vi "daqRead.vi"   [LabVIEW 2017]
doc: "From the DAQ card, reads into shared variables the external frame counter, the piezo monitor, and its differentiator. The acquisition is triggered by the Hamamatsu camera triggers. If daqSave is set to true, writes the values to file. \n\nThe acquisition loop stops with a daqStop (generally issued by the hamamatsuRead* VI) or, after a delay, with a generalStop."
uses:
  <vilib>/DAQmx/read.llb/DAQmx Read (Analog 1D DBL NChan 1Samp).vi
  <vilib>/DAQmx/read.llb/DAQmx Read (Counter U32 1Chan 1Samp).vi
  globalDevices.vi
  globalUtilities.vi
  <vilib>/DAQmx/miscellaneous.llb/DAQmx Fill In Error Info.vi
  <vilib>/DAQmx/read.llb/DAQmx Read (Analog DBL 1Chan 1Samp).vi
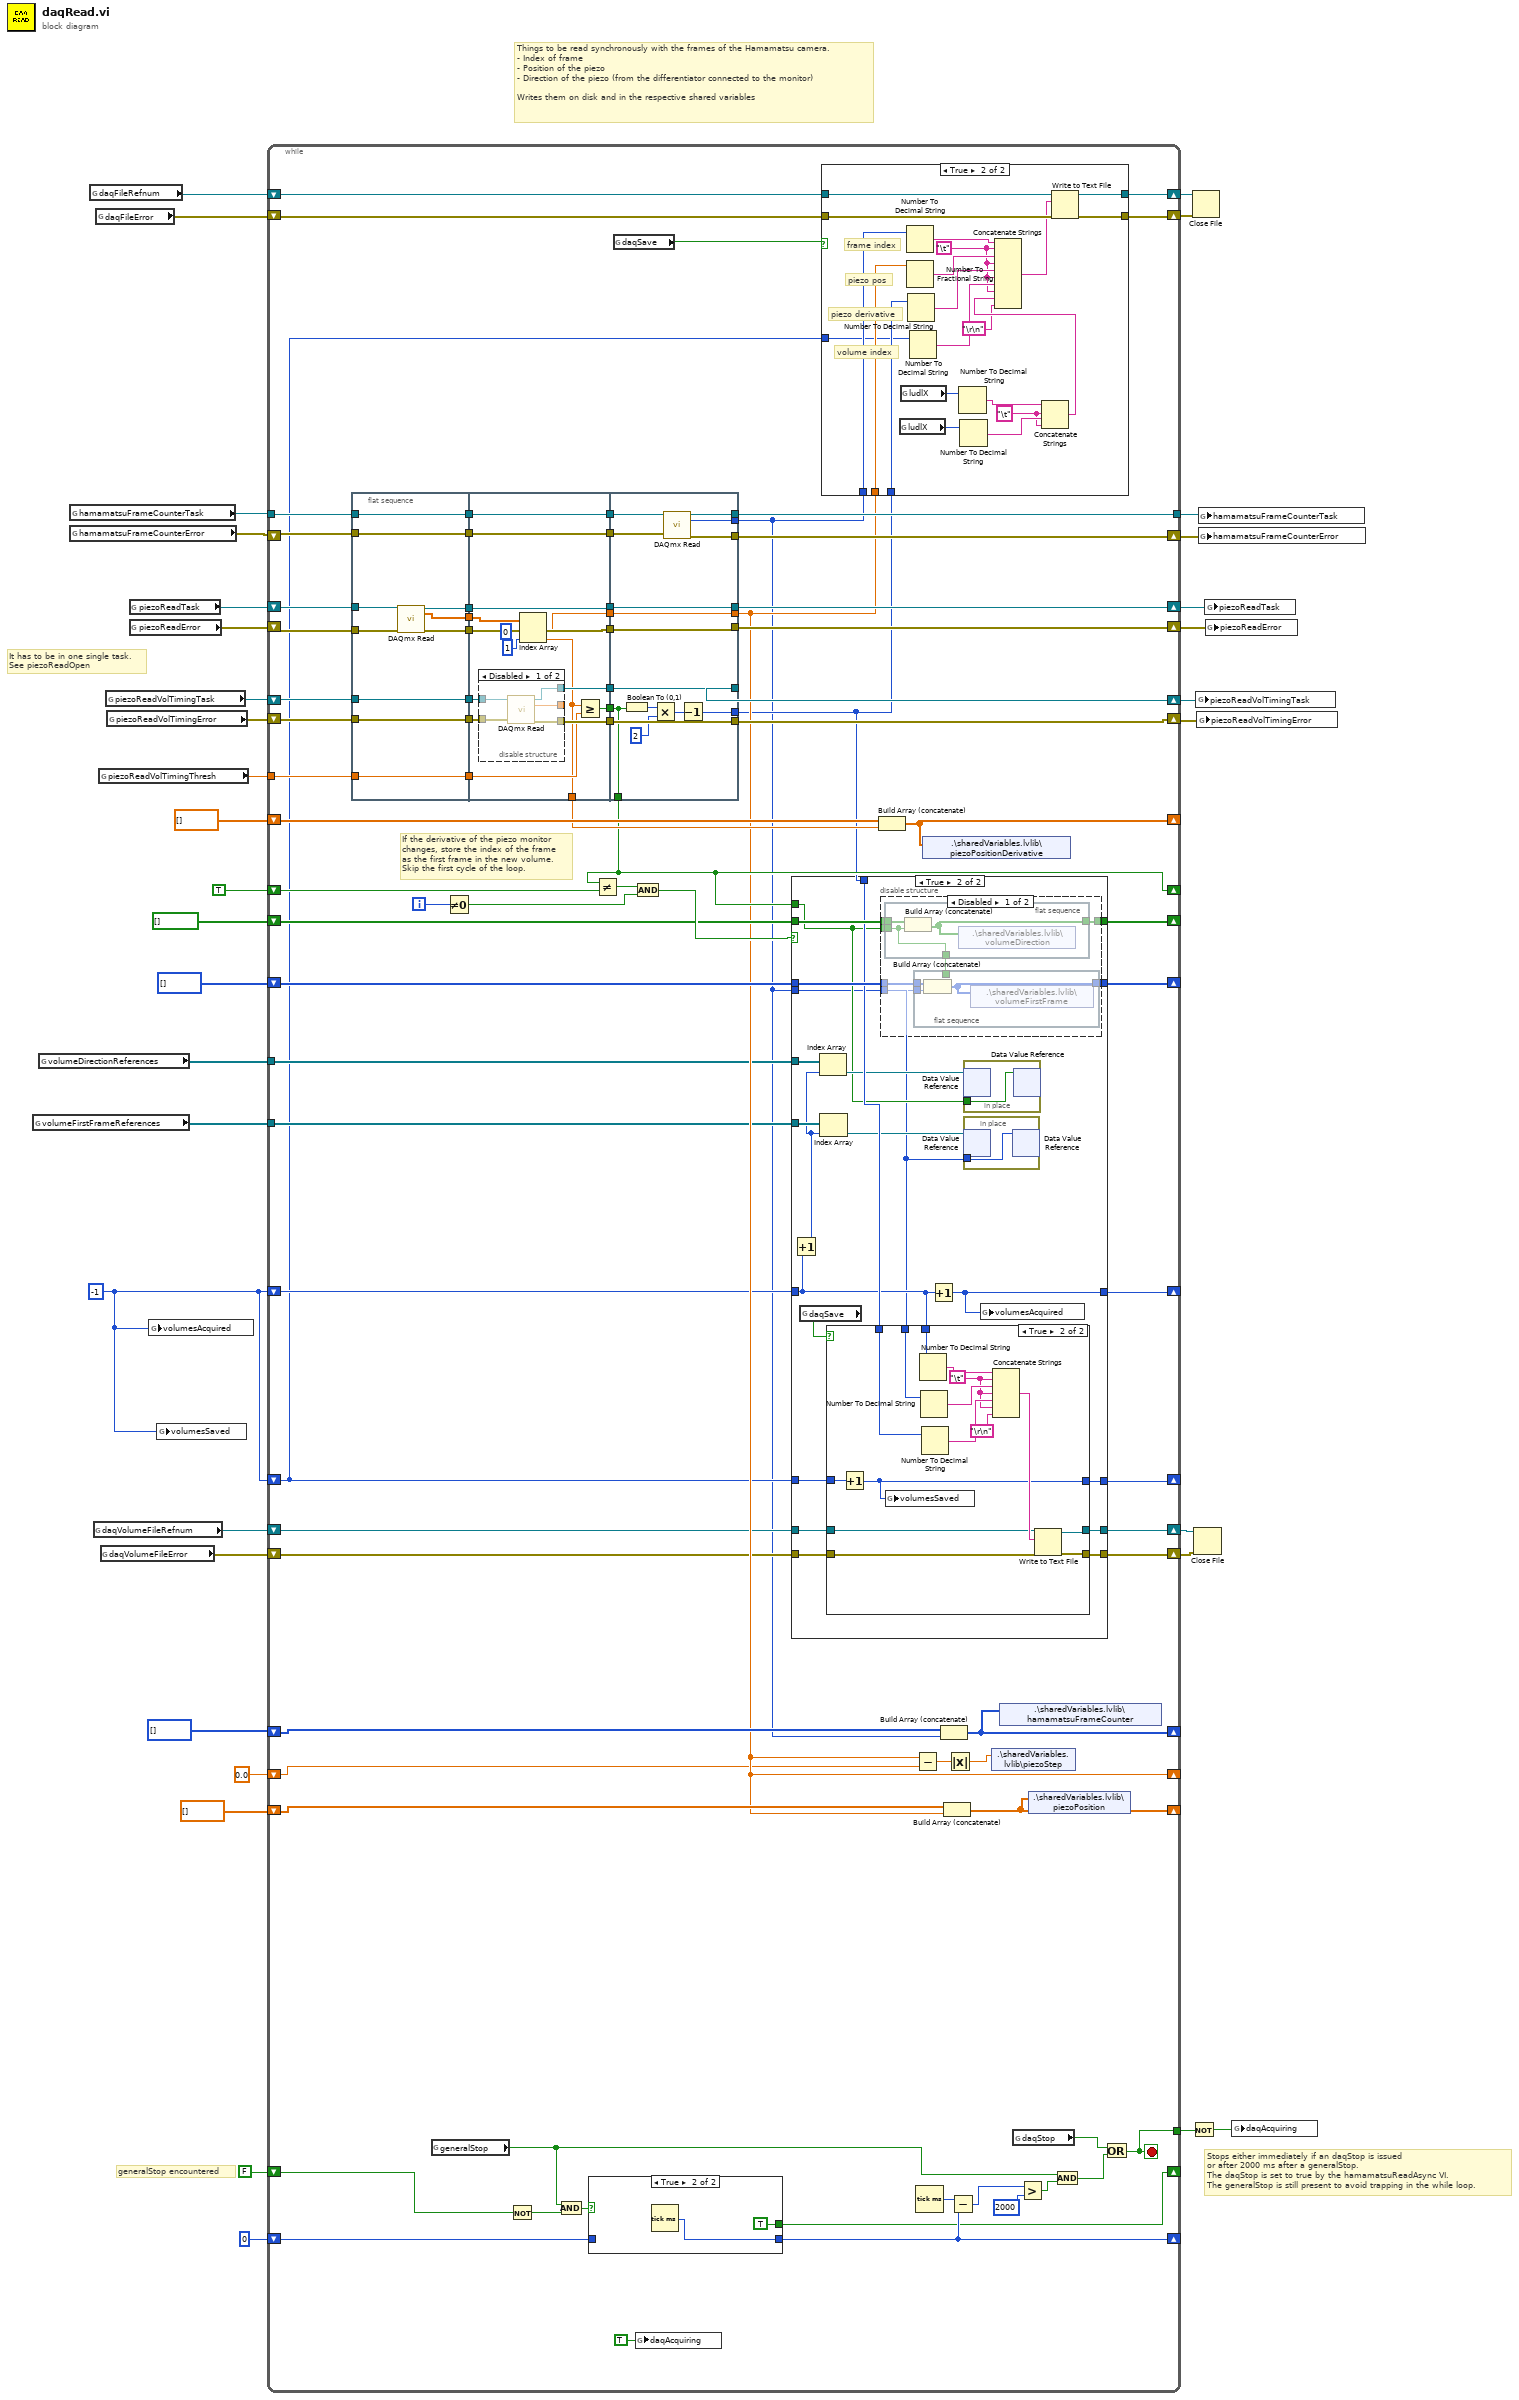
[diagram p0: block diagram]
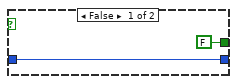
[diagram p5: hidden frame]
diagram:
  w1 = -1
  # "It has to be in one single task.\nSee piezoReadOpen"
  # "generalStop encountered"
  # "Stops either immediately if an daqStop is issued\nor after 2000 ms after a generalStop.\nThe daqStop is set to true by the hamamatsuReadAsync VI.\nThe generalStop is still present to avoid trapping in the while loop."
  # "Things to be read synchronously with the frames of the Hamamatsu camera.\n- Index of frame\n- Position of the piezo\n- Direction of the piezo (from the differentiator connected to the monitor)\n\nWrites them on disk and in the respective shared variables"
  n1 = global read "globalUtilities.vi" "volumeFirstFrameReferences"() -> (w2:refnum<data-value>[])
  n2 = global read "globalUtilities.vi" "volumeDirectionReferences"() -> (w3:refnum<data-value>[])
  n3 = global read "globalDevices.vi" "hamamatsuFrameCounterTask"() -> (w34:refnum<k21>)
  n4 = global read "globalDevices.vi" "hamamatsuFrameCounterError"() -> (w33:errorcluster)
  n5 = global read "globalDevices.vi" "daqFileRefnum"() -> (w14:refnum<file>)
  n6 = global read "globalDevices.vi" "daqVolumeFileRefnum"() -> (w7:refnum<file>)
  n7 = global read "globalDevices.vi" "daqFileError"() -> (w13:errorcluster)
  n8 = global read "globalDevices.vi" "piezoReadVolTimingThresh"() -> (w24:dbl)
  n9 = global read "globalDevices.vi" "daqVolumeFileError"() -> (w6:errorcluster)
  n10 = global read "globalDevices.vi" "piezoReadVolTimingTask"() -> (w26:refnum<k21>)
  n11 = global read "globalDevices.vi" "piezoReadVolTimingError"() -> (w25:errorcluster)
  n12 = global read "globalDevices.vi" "piezoReadTask"() -> (w35:refnum<k21>)
  n13 = global read "globalDevices.vi" "piezoReadError"() -> (w32:errorcluster)
  n14 = global write "globalUtilities.vi" "volumesAcquired"(w1) -> ()
  n15 = global write "globalUtilities.vi" "volumesSaved"(w1) -> ()
  n16 = while {
    tunnel: w34 -> [w115]
    shift-right: [w111] -> w16
    shift-left: w33 -> [w113]
    shift-right: [w109] -> w19
    shift-left: w32 -> [w112]
    shift-right: [w106] -> w29
    shift-left: w14 -> [w107]
    shift-right: [w103] -> _
    shift-left: u32[] [] -> [w105]
    shift-right: [w102] -> _
    shift-left: dbl[] [] -> [w104]
    shift-right: [w89] -> _
    shift-left: FALSE -> [w100]
    shift-right: [w94] -> _
    shift-left: u32 0 -> [w97]
    shift-right: [w85] -> w18
    shift-left: w25 -> [w87]
    tunnel: w24 -> [w84]
    shift-right: [w53] -> _
    shift-left: TRUE -> [w81]
    shift-right: [w76] -> _
    shift-left: u32[] [] -> [w77]
    shift-right: [w73] -> _
    shift-left: dbl[] [] -> [w75]
    shift-right: [w71] -> w20
    shift-left: w35 -> [w117]
    shift-right: [w69] -> w17
    shift-left: w26 -> [w88]
    tunnel: [w68] -> w15
    shift-right: [w58] -> w12
    shift-left: w13 -> [w108]
    tunnel: [w55] -> w11
    shift-right: [w52] -> _
    shift-left: bool[] [] -> [w54]
    shift-right: [w51] -> _
    shift-left: 0.0 -> [w50]
    shift-right: [w44] -> w4
    shift-left: w6 -> [w46]
    shift-right: [w45] -> w5
    shift-left: w7 -> [w47]
    shift-right: [w42] -> _
    shift-left: w1 -> [w43]
    tunnel: w3 -> [w40]
    tunnel: w2 -> [w39]
    shift-right: [w38] -> _
    shift-left: w1 -> [w37]
    i -> [w82]
    stop <- w55 stop-if-true
    # "If the derivative of the piezo monitor\nchanges, store the index of the frame\nas the first frame in the new volume.\nSkip the first cycle of the loop."
    n17 = flat-sequence {
      tunnel: w84 -> [w210]
      tunnel: w87 -> [w211]
      tunnel: w88 -> [w212]
      tunnel: w113 -> [w213]
      tunnel: w112 -> [w208]
      tunnel: w115 -> [w214]
      tunnel: w117 -> [w209]
      tunnel: [w214] -> w67
      tunnel: [w213] -> w66
      tunnel: [w212] -> w65
      tunnel: [w211] -> w64
      tunnel: [w210] -> w63
      tunnel: [w207] -> w62
      tunnel: [w206] -> w61
      tunnel: [w205] -> w59
      tunnel: [w229] -> w116
      tunnel: [w228] -> w114
      tunnel: [w220] -> w110
      tunnel: [w225] -> w86
      tunnel: [w223] -> w83
      tunnel: [w215] -> w74
      tunnel: [w221] -> w72
      tunnel: [w222] -> w70
      tunnel: w67 -> [w229]
      tunnel: w66 -> [w228]
      tunnel: w65 -> [w227]
      tunnel: w64 -> [w226]
      tunnel: w63 -> [w224]
      tunnel: w62 -> [w221]
      tunnel: w61 -> [w219]
      tunnel: [w216] -> w60
      tunnel: w59 -> [w220]
      tunnel: w116 -> [w249]
      tunnel: w114 -> [w248]
      tunnel: [w247] -> w51
      tunnel: [w246] -> w36
      tunnel: [w245] -> w111
      tunnel: [w244] -> w109
      tunnel: w110 -> [w244]
      tunnel: [w243] -> w85
      tunnel: w86 -> [w243]
      tunnel: w83 -> [w238]
      tunnel: [w239] -> w41
      tunnel: [w238] -> w53
      tunnel: w72 -> [w237]
      tunnel: [w237] -> w71
      tunnel: w70 -> [w236]
      tunnel: [w236] -> w69
      tunnel: [w235] -> w68
      tunnel: w60 -> [w247]
      frame #0 {
        n18 = call-poly <vilib>:"DAQmx Read.vi"("task/channels in"=w209, "error in"=w208) -> ("task out"=w207:refnum<k21>, "data"=w206:dbl[], "error out"=w205:errorcluster)  [unwired: 11 in]
      }
      frame #1 {
        n19 = disable-structure shown="Disabled" {
          disable-tunnel: w227 -> [w234 _]
          disable-tunnel: w226 -> [w233 _]
          disable-tunnel: [w232 _] -> w225
          disable-tunnel: [w231 _] -> _
          disable-tunnel: [w230 _] -> w222
          frame Disabled {
            n20 = call-poly <vilib>:"DAQmx Read.vi"("task/channels in"=w234, "error in"=w233) -> ("task out"=w230:refnum<k21>, "data"=w231:dbl, "error out"=w232:errorcluster)  [unwired: 11 in]
          }
          frame Enabled {
          }
        }
        n21 = Index Array(array=w219, index #1=0 ("index"), index #2=1 ("index")) -> (element #1=w216:dbl, element #2=w215:dbl)
        n22 = Greater Or Equal?(x=w215, y=w224) -> (x >= y?=w223:bool)
      }
      frame #2 {
        n23 = Boolean To (0,1)(Boolean=w238) -> (0, 1=w242:i16)
        n24 = Multiply(x=w242, y=i16 2) -> (x*y=w240:i16)
        n25 = call-poly <vilib>:"DAQmx Read.vi"("task/channels in"=w249, "error in"=w248) -> ("task out"=w235:refnum<k21>, "data"=w246:u32, "error out"=w245:errorcluster)  [unwired: 11 in]
        n26 = Decrement(x=w240) -> (x-1=w239:i16)
      }
    }
    n27 = global read "globalUtilities.vi" "generalStop"() -> (w96:bool)
    n28 = Not Equal To 0?(x=w82) -> (x != 0?=w79:bool)
    n29 = Not(x=w100) -> (.not. x?=w98:bool)
    n30 = And(x=w96, y=w98) -> (x .and. y?=w99:bool)
    n31 = case shown="True" w99 {
      tunnel: w97 -> [w179 _]
      tunnel: [w179 w181] -> w94
      tunnel: [FALSE TRUE] -> w89
      frame False {
      }
      frame True {
        n32 = Tick Count (ms)() -> (millisecond timer value=w181:u32)
      }
    }
    n33 = Not Equal?(x=w53, y=w81) -> (x != y?=w80:bool)
    n34 = global read "globalUtilities.vi" "daqSave"() -> (w101:bool)
    n35 = And(x=w80, y=w79) -> (x .and. y?=w78:bool)
    n36 = global write "globalUtilities.vi" "daqAcquiring"(TRUE ("daqAcquiring")) -> ()
    n37 = case shown="True" w78 {
      tunnel: w77 -> [w123 w144]
      tunnel: w36 -> [_ w127]
      tunnel: [w123 w143] -> w76
      tunnel: w54 -> [w122 w142]
      tunnel: w53 -> [_ w131]
      tunnel: [w122 w141] -> w52
      tunnel: w47 -> [w120 w139]
      tunnel: w46 -> [w119 w138]
      tunnel: [w120 w137] -> w45
      tunnel: [w119 w136] -> w44
      tunnel: w43 -> [w121 w129]
      tunnel: [w121 w134] -> w42
      tunnel: w41 -> [_ w135]
      tunnel: w40 -> [_ w133]
      tunnel: w39 -> [_ w130]
      tunnel: w37 -> [w118 w125]
      tunnel: [w118 w124] -> w38
      frame False {
      }
      frame True {
        n38 = Increment(x=w129) -> (x+1=w126:i32)
        n39 = global read "globalUtilities.vi" "daqSave"() -> (w140:bool)
        n40 = Index Array(array=w133, index=w126) -> (element=w132:refnum<data-value>)
        n41 = Index Array(array=w130, index=w126) -> (element=w128:refnum<data-value>)
        n42 = case shown="True" w140 {
          tunnel: w139 -> [w162 w168]
          tunnel: w138 -> [w161 w167]
          tunnel: [w162 w166] -> w137
          tunnel: [w161 w165] -> w136
          tunnel: w129 -> [_ w177]
          tunnel: w127 -> [_ w176]
          tunnel: w135 -> [_ w175]
          tunnel: w125 -> [w160 w164]
          tunnel: [w160 w163] -> w124
          frame False {
          }
          frame True {
            w171 = "\t"
            n43 = Increment(x=w164) -> (x+1=w163:i32)
            n44 = global write "globalUtilities.vi" "volumesSaved"(w163) -> ()
            n45 = Number To Decimal String(number=w177) -> (decimal integer string=w174:string)  [unwired: 1 in]
            n46 = Number To Decimal String(number=w176) -> (decimal integer string=w173:string)  [unwired: 1 in]
            n47 = Number To Decimal String(number=w175) -> (decimal integer string=w172:string)  [unwired: 1 in]
            n48 = Concatenate Strings(w174, w171, w173, w171, w172, w171, "\r\n") -> (w169:string)
            n49 = Write to Text File(file (use dialog)=w168, text=w169, error in=w167) -> (refnum out=w166:refnum<file>, error out=w165:errorcluster)  [unwired: 1 in, 1 out]
          }
        }
        n50 = disable-structure shown="Disabled" {
          disable-tunnel: w144 -> [w151 _]
          disable-tunnel: [w150 _] -> w143
          disable-tunnel: w142 -> [w149 _]
          disable-tunnel: [w148 _] -> w141
          disable-tunnel: w131 -> [w146 _]
          disable-tunnel: w127 -> [w145 _]
          frame Disabled {
            n51 = flat-sequence {
              tunnel: w149 -> [w157]
              tunnel: [w156] -> w148
              tunnel: w146 -> [w155]
              tunnel: [w155] -> w147
              frame #0 {
                n52 = Build Array (concatenate)(w157, w155) -> (w156:bool[])
                n53 = shared-variable ".\\sharedVariables.lvlib\\volumeDirection"(w156) -> ()  [unwired: 1 in, 1 out]
              }
            }
            n54 = flat-sequence {
              tunnel: w151 -> [w154]
              tunnel: [w153] -> w150
              tunnel: w145 -> [w152]
              tunnel: w147 -> [_]
              frame #0 {
                n55 = Build Array (concatenate)(w154, w152) -> (w153:u32[])
                n56 = shared-variable ".\\sharedVariables.lvlib\\volumeFirstFrame"(w153) -> ()  [unwired: 1 in, 1 out]
              }
            }
          }
          frame Enabled {
          }
        }
        n57 = Increment(x=w129) -> (x+1=w134:i32)
        n58 = in-place {
          in-place-border: w131 -> [w159]
          n59 = in-place-dvr #1(w132) -> ()  [unwired: 2 out]
          n60 = in-place-dvr #1(w159) -> ()  [unwired: 2 out]
        }
        n61 = in-place {
          in-place-border: w127 -> [w158]
          n62 = in-place-dvr #2(w128) -> ()  [unwired: 2 out]
          n63 = in-place-dvr #2(w158) -> ()  [unwired: 2 out]
        }
        n64 = global write "globalUtilities.vi" "volumesAcquired"(w134) -> ()
      }
    }
    n65 = case shown="True" w101 {
      tunnel: w108 -> [w182 w202]
      tunnel: w107 -> [w183 w200]
      tunnel: [w183 w199] -> w106
      tunnel: [w182 w198] -> w58
      tunnel: w36 -> [_ w197]
      tunnel: w51 -> [_ w196]
      tunnel: w41 -> [_ w194]
      tunnel: w37 -> [_ w193]
      frame False {
      }
      frame True {
        w187 = "\t" ("string")
        w186 = "\t"
        # "volume index"
        # "piezo derivative"
        # "piezo pos"
        # "frame index"
        n66 = global read "globalDevices.vi" "ludlX"() -> (w188:i32)
        n67 = global read "globalDevices.vi" "ludlX"() -> (w189:i32)
        n68 = Number To Decimal String(number=w197) -> (decimal integer string=w204:string)  [unwired: 1 in]
        n69 = Number To Fractional String(number=w196) -> (F-format string=w203:string)  [unwired: 3 in]
        n70 = Number To Decimal String(number=w194) -> (decimal integer string=w195:string)  [unwired: 1 in]
        n71 = Number To Decimal String(number=w193) -> (decimal integer string=w192:string)  [unwired: 1 in]
        n72 = Number To Decimal String(number=w189) -> (decimal integer string=w190:string)  [unwired: 1 in]
        n73 = Number To Decimal String(number=w188) -> (decimal integer string=w191:string)  [unwired: 1 in]
        n74 = Concatenate Strings(w190, w187, w191, w187) -> (w185:string)
        n75 = Concatenate Strings(w204, w186, w203, w186, w195, w186, w192, w186, w185, "\r\n") -> (w201:string)
        n76 = Write to Text File(file (use dialog)=w200, text=w201, error in=w202) -> (refnum out=w199:refnum<file>, error out=w198:errorcluster)  [unwired: 1 in, 1 out]
      }
    }
    n77 = Build Array (concatenate)(w75, w74) -> (w73:dbl[])
    n78 = Subtract(x=w51, y=w50) -> (x-y=w49:dbl)
    n79 = Tick Count (ms)() -> (millisecond timer value=w95:u32)
    n80 = shared-variable ".\\sharedVariables.lvlib\\piezoPositionDerivative"(w73) -> ()  [unwired: 1 in, 1 out]
    n81 = Build Array (concatenate)(w105, w36) -> (w103:u32[])
    n82 = Build Array (concatenate)(w104, w51) -> (w102:dbl[])
    n83 = Absolute Value(x=w49) -> (abs(x)=w48:dbl)
    n84 = Subtract(x=w95, y=w94) -> (x-y=w93:u32)
    n85 = shared-variable ".\\sharedVariables.lvlib\\piezoStep"(w48) -> ()  [unwired: 1 in, 1 out]
    n86 = shared-variable ".\\sharedVariables.lvlib\\hamamatsuFrameCounter"(w103) -> ()  [unwired: 1 in, 1 out]
    n87 = global read "globalUtilities.vi" "daqStop"() -> (w56:bool)
    n88 = Greater?(x=w93, y=u32 2000) -> (0:w91:bool)
    n89 = shared-variable ".\\sharedVariables.lvlib\\piezoPosition"(w102) -> ()  [unwired: 1 in, 1 out]
    n90 = And(x=w96, y=w91) -> (x .and. y?=w90:bool)
    n91 = Or(x=w56, y=w90) -> (x .or. y?=w55:bool)
  }
  n92 = Not(x=w11) -> (.not. x?=w10:bool)
  n93 = Close File(refnum=w29, error in=w12) -> ()  [unwired: 2 out]
  n94 = Close File(refnum=w5, error in=w4) -> ()  [unwired: 2 out]
  n95 = global write "globalDevices.vi" "piezoReadVolTimingTask"(w17) -> ()
  n96 = global write "globalDevices.vi" "piezoReadVolTimingError"(w18) -> ()
  n97 = global write "globalDevices.vi" "hamamatsuFrameCounterTask"(w15) -> ()
  n98 = global write "globalDevices.vi" "hamamatsuFrameCounterError"(w16) -> ()
  n99 = global write "globalDevices.vi" "piezoReadTask"(w20) -> ()
  n100 = global write "globalDevices.vi" "piezoReadError"(w19) -> ()
  n101 = global write "globalUtilities.vi" "daqAcquiring"(w10) -> ()
